vi "Communication Bus Template.Async.vi"(10 "Parameters":variant, 11 "Process":refnum<class "Process.lvclass">) -> ()   [LabVIEW 2020, in "Communication Bus Template Engine.lvlib" / "Custom Device.lvlib"]
uses:
  Custom Device.lvlib
  <vilib>/NI/NIVS Inline Async API/_VS Inline Async API/Process/Process.lvclass
  <vilib>/NI/NIVS Inline Async API/_Data Access Engine/Data Access Engine/Data Access Engine.lvclass
  Asynchronous Execution Unit Runtime Information.ctl
  <vilib>/NI/NIVS Inline Async API/_Data Access Engine/Data Access Engine/Methods/Read.Lookup.vi
  <vilib>/NI/NIVS Inline Async API/_Data Access Engine/Data Access Engine/Methods/Write.Lookup.vi
  <vilib>/NI/NIVS Inline Async API/_Data Access Engine/Data Access Engine/Methods/Write.Data.vi
  <vilib>/NI/NIVS Inline Async API/_Data Access Engine/Data Access Engine/Methods/Read.Data.vi
  Interfaces/Execution Unit/Execution Unit.lvclass
  Interfaces/Shared Resources/Shared Resources.lvclass
  Asynchronous Process Parameters.ctl
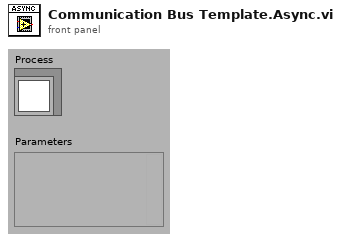
[diagram p1: front panel]
types:
  T1 = typedef "Communication Bus Template Engine.lvlib/Custom Device.lvlib/Asynchronous Process Parameters.ctl" = cluster{"Asynchronous Execution Unit Runtime Information":T2, "shared resources":refnum<class "Shared Resources.lvclass">}
  T2 = typedef "Communication Bus Template Engine.lvlib/Custom Device.lvlib/Asynchronous Execution Unit Runtime Information.ctl" = cluster{"Execution Unit":refnum<class "Execution Unit.lvclass">, "Incoming Channel Group Name":string, "Outgoing Channel Group Name":string}
  T3 = typedef "Data Access Engine.lvlib/Data Access Engine.lvclass/Write.DVR.ctl" = refnum<data-value>
  T4 = typedef "Data Access Engine.lvlib/Data Access Engine.lvclass/Read.DVR.ctl" = refnum<data-value>
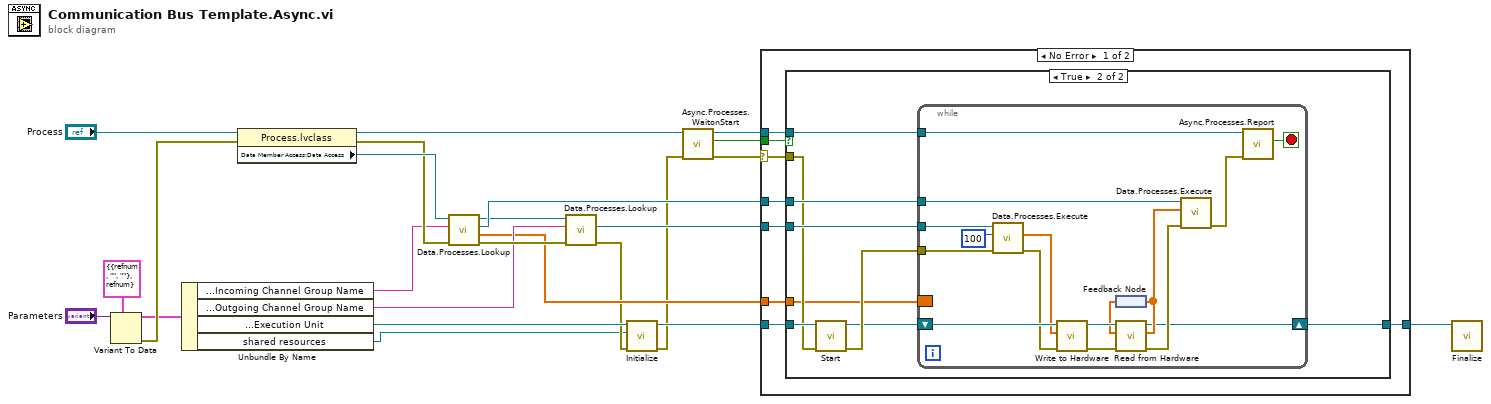
[diagram p0: block diagram]
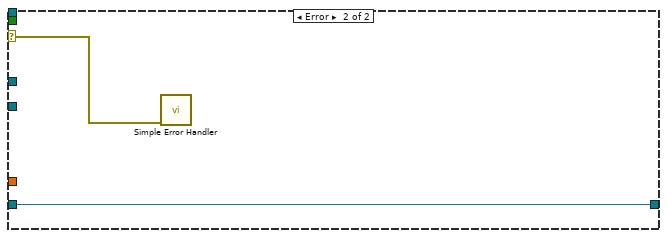
[diagram p3: hidden frame]
diagram:
  n1 = Variant To Data(type=T1 {"Asynchronous Execution Unit Runtime Information"={"Execution Unit"=refnum, "Incoming Channel Group Name"="", "Outgoing Channel Group Name"=""}, "shared resources"=refnum} ("Asynchronous Process Parameters"), Variant="Parameters") -> (data=w10:T1, error out=w11:errorcluster)  [unwired: 1 in]
  n2 = Unbundle By Name(w10) -> ("Asynchronous Execution Unit Runtime Information.Incoming Channel Group Name"=w9:string, "Asynchronous Execution Unit Runtime Information.Outgoing Channel Group Name"=w8:string, "Asynchronous Execution Unit Runtime Information.Execution Unit"=w6:refnum<class "Execution Unit.lvclass">, "shared resources"=w1:refnum<class "Shared Resources.lvclass">)
  n3 = property class="Process.lvclass"(reference="Process", error in=w11) -> (reference out=w16:refnum<class "Process.lvclass">, error out=w14:errorcluster, "Data Member Access:Data Access"=w15:refnum<class "Data Access Engine.lvclass">)
  n4 = call-poly <vilib>:"Data.Processes.Lookup.vi"("error in (no error)"=w14, "Name"=w9, "Data Access API in"=w15) -> ("error out"=w20:errorcluster, "Initial Values"=w7:dbl[], "Ref"=w19:T3, "Data Access API out"=w18:refnum<class "Data Access Engine.lvclass">)  [unwired: 5 in]
  n5 = call-poly <vilib>:"Data.Processes.Lookup.vi"("error in (no error)"=w20, "Name"=w8, "Data Access API in"=w18) -> ("error out"=w4:errorcluster, "Ref"=w21:T4)  [unwired: 5 in, 2 out]
  n6 = call-dynamic "Initialize.vi"("error in (no error)"=w4, "shared resources"=w1, "Execution Unit in"=w6) -> ("error out"=w3:errorcluster, "Execution Unit out"=w5:refnum<class "Execution Unit.lvclass">)  [unwired: 7 in]
  n7 = call <vilib>:"Async.Processes.WaitonStart.vi"("error in (no error)"=w3, "Process"=w16) -> ("error out"=w22:errorcluster, "Execute"=w24:bool, "Process out"=w23:refnum<class "Process.lvclass">)  [unwired: 7 in]
  n8 = case shown="No Error" w22 {
    selector: w22 -> [w28 w60]
    tunnel: w24 -> [w32 _]
    tunnel: w23 -> [w31 _]
    tunnel: w19 -> [w30 _]
    tunnel: w21 -> [w29 _]
    tunnel: w7 -> [w27 _]
    tunnel: w5 -> [w26 w59]
    tunnel: [w25 w59] -> w2
    frame No Error {
      n9 = case shown="True" w32 {
        tunnel: w28 -> [_ w38]
        tunnel: w31 -> [_ w40]
        tunnel: w29 -> [_ w42]
        tunnel: w30 -> [_ w41]
        tunnel: w27 -> [_ w35]
        tunnel: w26 -> [w33 w39]
        tunnel: [w33 w34] -> w25
        frame False {
        }
        frame True {
          n10 = call-dynamic "Start.vi"("error in (no error)"=w38, "Execution Unit in"=w39) -> ("error out"=w37:errorcluster, "Execution Unit out"=w36:refnum<class "Execution Unit.lvclass">)  [unwired: 8 in]
          n11 = while {
            tunnel: w37 -> [w54]
            tunnel: w40 -> [w58]
            tunnel: w42 -> [w56]
            tunnel: w41 -> [w55]
            border: w35 -> [_]
            shift-right: [w43] -> w34
            shift-left: w36 -> [w52]
            stop <- w57 stop-if-true
            n12 = call-poly <vilib>:"Data.Processes.Execute.vi"("error in (no error)"=w54, "timeout ms"=100, "Ref"=w56) -> ("error out"=w49:errorcluster, "Values"=w50:dbl[])  [unwired: 6 in, 1 out]
            n13 = call-dynamic "Write to Hardware.vi"("error in (no error)"=w49, "Values in"=w50, "Execution Unit in"=w52) -> ("error out"=w48:errorcluster, "Execution Unit out"=w51:refnum<class "Execution Unit.lvclass">)  [unwired: 6 in, 1 out]
            n14 = feedback #1() -> (w45:dbl[])
            n15 = call-dynamic "Read from Hardware.vi"("error in (no error)"=w48, "Values in"=w45, "Execution Unit in"=w51) -> ("error out"=w47:errorcluster, "Values out"=w44:dbl[], "Execution Unit out"=w43:refnum<class "Execution Unit.lvclass">)  [unwired: 6 in]
            n16 = feedback-in #1(w44) -> ()
            n17 = call-poly <vilib>:"Data.Processes.Execute.vi"("error in (no error)"=w47, "Values"=w44, "Ref"=w55) -> ("error out"=w46:errorcluster)  [unwired: 8 in]
            n18 = call <vilib>:"Async.Processes.Report.vi"("Error"=w46, "Process in"=w58) -> ("Stop"=w57:bool)  [unwired: 8 in, 1 out]
          }
        }
      }
    }
    frame Error {
      n19 = call <vilib>:"Simple Error Handler.vi"("error in (no error)"=w60) -> ()  [unwired: 4 in, 5 out]
    }
  }
  n20 = call-dynamic "Finalize.vi"("Execution Unit in"=w2) -> ()  [unwired: 9 in, 2 out]
